vi "Set value attributes.vi"(7 "item ref":refnum<vi>, 8 "error in (no error)":errorcluster, 10 "Value string":string, 11 "Session In":T1) -> (0 "error out":errorcluster, 3 "IMAQdx Session":T1)   [LabVIEW 2016]
uses:
  <vilib>/userdefined/High Color/IMAQdx.ctl
  <vilib>/Utility/miscctls.llb/LVMinMaxIncTypeDef.ctl
  <resource>/objmgr/imaqdx.rc
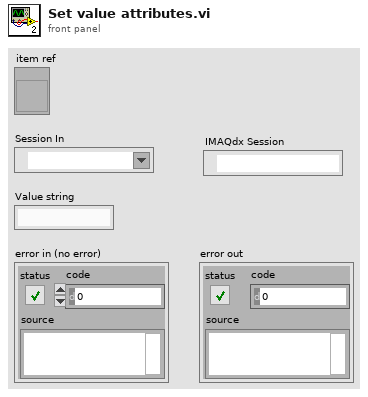
[diagram p1: front panel]
types:
  T1 = typedef "IMAQdx.ctl" = refnum<k21>
  T2 = typedef "LVMinMaxIncTypeDef.ctl" = cluster{"Minimum":dbl, "Maximum":dbl, "Increment":dbl}
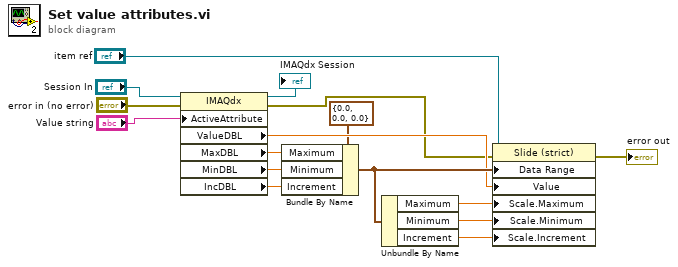
[diagram p0: block diagram]
diagram:
  n1 = property class="IMAQdx"(reference="Session In", error in="error in (no error)", "ActiveAttribute"="Value string") -> (reference out=→"IMAQdx Session":T1, error out=w1:errorcluster, "ValueDBL"=w9:dbl, "MaxDBL"=w6:dbl, "MinDBL"=w7:dbl, "IncDBL"=w8:dbl)
  n2 = Bundle By Name(cluster=T2 {"Minimum"=0.0, "Maximum"=0.0, "Increment"=0.0} ("Data Entry Limits"), "Maximum"=w6, "Minimum"=w7, "Increment"=w8) -> (w12:T2)
  n3 = Unbundle By Name(w12) -> ("Maximum"=w13:dbl, "Minimum"=w14:dbl, "Increment"=w15:dbl)
  n4 = property class="Slide (strict)"(reference="item ref", error in=w1, "Data Range"=w12, "Value"=w9, "Scale.Maximum"=w13, "Scale.Minimum"=w14, "Scale.Increment"=w15) -> (error out=→"error out":errorcluster)  [unwired: 1 out]
